vi "Kalman_Filter_Setter_Online.vi"(8 "error in (no error)":errorcluster, 10 "KF":T1, 11 "Kalman_Filter in":refnum<class "Kalman_Filter.lvclass">) -> (0 "error out":errorcluster, 3 "Kalman_Filter out":refnum<class "Kalman_Filter.lvclass">)   [LabVIEW 2021, in "Kalman_Filter.lvclass"]
uses:
  Kalman_Filter.lvclass
  Kalman_Filter.lvclass/Kalman_Filter.ctl
  <vilib>/Analysis/7linalg.llb/Real Matrix Exp.vi
  <vilib>/Analysis/Matrix/Numeric/Absolute Value/Absolute Value - RM.vi
  <vilib>/Analysis/NI_AALBase.lvlib
  <vilib>/Analysis/Matrix/NI_Matrix.lvlib
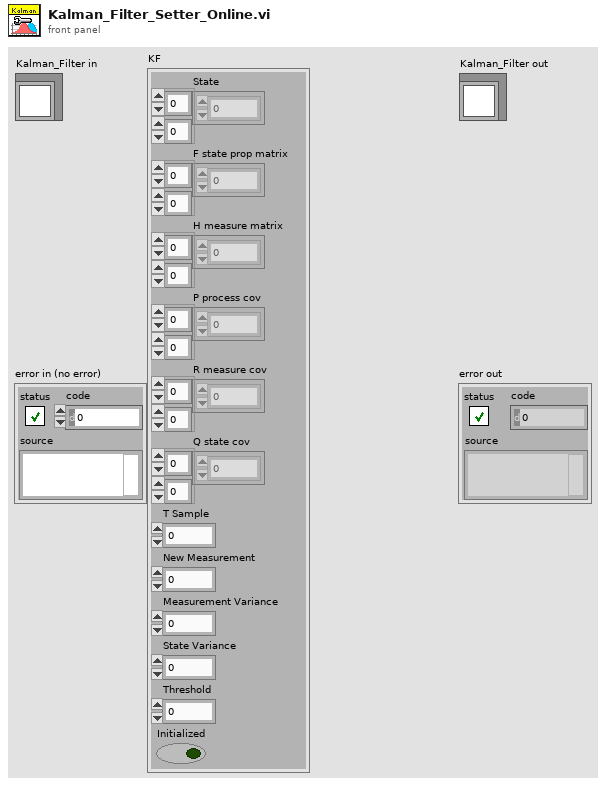
[diagram p1: front panel]
types:
  T1 = cluster{"State":dbl[][], "F state prop matrix":dbl[][], "H measure matrix":dbl[][], "P process cov":dbl[][], "R measure cov":dbl[][], "Q state cov":dbl[][], "T Sample":dbl, "New Measurement":dbl, "Measurement Variance":dbl, "State Variance":dbl, "Threshold":dbl, "Initialized":bool}
  T2 = typedef "NI_Matrix.lvlib/RealMatrix.ctl" = dbl[][]
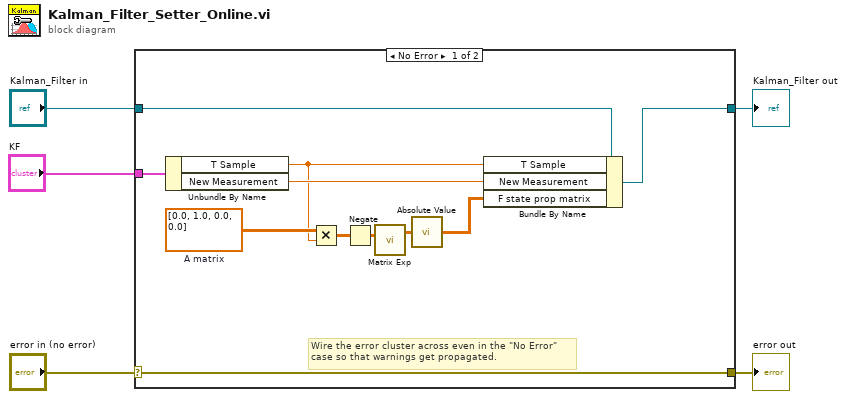
[diagram p0: block diagram]
diagram:
  n1 = case shown="No Error" "error in (no error)" {
    selector: "error in (no error)" -> [w16 w18]
    tunnel: [w16 w18] -> w4
    tunnel: [w14 w17] -> w2
    tunnel: "Kalman_Filter in" -> [w15 w17]
    tunnel: "KF" -> [w13 _]
    frame No Error {
      w9 = dbl[][] [[0.0, 1.0], [0.0, 0.0]]  # A matrix
      # "Wire the error cluster across even in the \"No Error\"\ncase so that warnings get propagated."
      n2 = Unbundle By Name(w13) -> ("T Sample"=w7:dbl, "New Measurement"=w12:dbl)
      n3 = Multiply(x=w9, y=w7) -> (x*y=w10:dbl[][])
      n4 = Negate(x=w10) -> (-x=w11:dbl[][])
      n5 = call-poly <vilib>:"Matrix Exp.vi"("Input Matrix"=w11) -> ("Matrix Exp"=w8:T2)  [unwired: 1 in, 1 out]
      n6 = call-poly <vilib>:"Absolute Value.vi"("Real Matrix A"=w8) -> ("|A|"=w6:T2)
      n7 = Bundle By Name(cluster=w15, "T Sample"=w7, "New Measurement"=w12, "F state prop matrix"=w6) -> (w14:refnum<class "Kalman_Filter.lvclass">)
    }
    frame Error {
    }
  }
  "error out" <- w4
  "Kalman_Filter out" <- w2
